vi "testSerial.vi"() -> ()   [LabVIEW 2013]
uses:
  <vilib>/Instr/_visa.llb/VISA Configure Serial Port (Instr).vi
panel:
  out "count":u32
  out "Read":string
  in  "stop":bool
  in  "OK Button":bool
  in  "Write":string
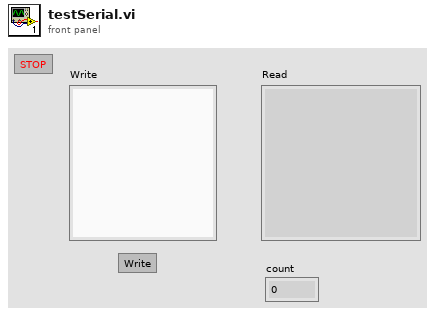
[diagram p1: front panel]
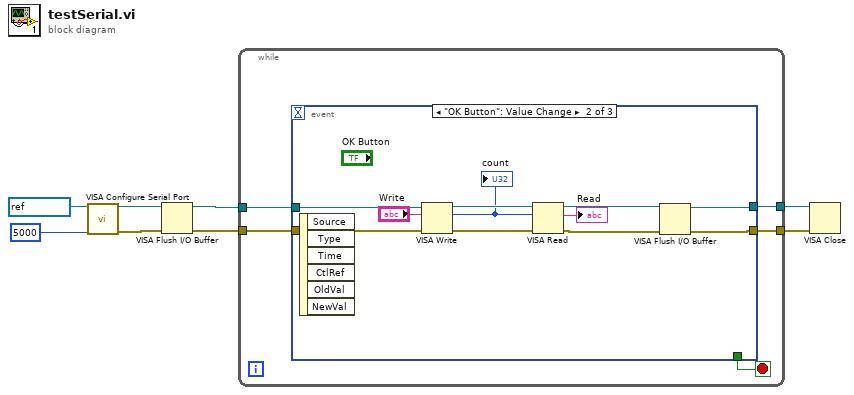
[diagram p0: block diagram]
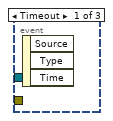
[diagram p2: hidden frame]
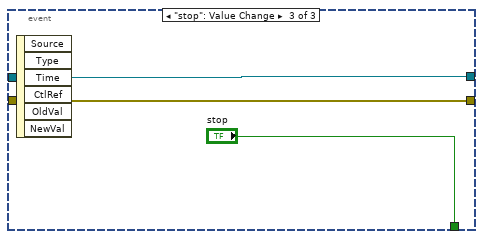
[diagram p3: hidden frame]
diagram:
  n1 = call-poly "VISA Configure Serial Port"("VISA resource name"=refnum<visa-resource-name> "COM3", "timeout (10sec)"=u32 5000) -> ("VISA resource name out"=w1:refnum<visa-resource-name>, "error out"=w2:errorcluster)  [unwired: 12 in]
  n2 = VISA Flush I/O Buffer(VISA resource name=w1, error in (no error)=w2) -> (VISA resource name out=w4:refnum<visa-resource-name>, error out=w3:errorcluster)  [unwired: 1 in]
  n3 = while {
    tunnel: w4 -> [w13]
    tunnel: w3 -> [w12]
    tunnel: [w11] -> w6
    tunnel: [w10] -> w5
    stop <- w9 stop-if-true
    n4 = event shown="[1] \"OK Button\": Value Change" {
      selector: _ -> [_ _ _]
      dyn-events: _ -> [_ _ _]
      timeout: _ -> [_ _ _]
      tunnel: w13 -> [_ w24 w26]
      tunnel: w12 -> [_ w22 w25]
      tunnel: [_ w16 w25] -> w11
      tunnel: [_ w17 w26] -> w10
      tunnel: [_ _ "stop"] -> w9
      event Timeout {
        n5 = event-data() -> ()  [unwired: 1 in, 3 out]
      }
      event "OK Button": Value Change {
        n6 = event-data() -> ()  [unwired: 1 in, 6 out]
        n7 = VISA Write(VISA resource name=w24, write buffer="Write", error in (no error)=w22) -> (VISA resource name out=w21:refnum<visa-resource-name>, return count=w18:u32, error out=w20:errorcluster)
        "count" <- w18
        n8 = VISA Read(VISA resource name=w21, byte count=w18, error in (no error)=w20) -> (VISA resource name out=w14:refnum<visa-resource-name>, read buffer=→"Read":string, error out=w15:errorcluster)  [unwired: 1 out]
        n9 = VISA Flush I/O Buffer(VISA resource name=w14, error in (no error)=w15) -> (VISA resource name out=w17:refnum<visa-resource-name>, error out=w16:errorcluster)  [unwired: 1 in]
      }
      event "stop": Value Change {
        n10 = event-data() -> ()  [unwired: 1 in, 6 out]
      }
    }
  }
  n11 = VISA Close(VISA resource name=w5, error in (no error)=w6) -> ()  [unwired: 1 out]
